vi "Read Timeout Message Priority.vi"(8 "error in (no error)":errorcluster, 11 "IEventHandler in":refnum<class "IEventHandler.lvclass">) -> (0 "error out":errorcluster, 2 "Timeout Message Priority":T1=enum."Normal", 3 "IEventHandler out":refnum<class "IEventHandler.lvclass">)   [LabVIEW 2015, in "ActorEvents.lvlib" / "IEventHandler.lvclass"]
uses:
  IEventHandler.lvclass
  <vilib>/ActorFramework/Message Enqueuer/Message Priority.ctl
  IEventHandler.lvclass/IEventHandler.ctl
  <vilib>/ActorFramework/Message Enqueuer/Message Enqueuer.lvclass
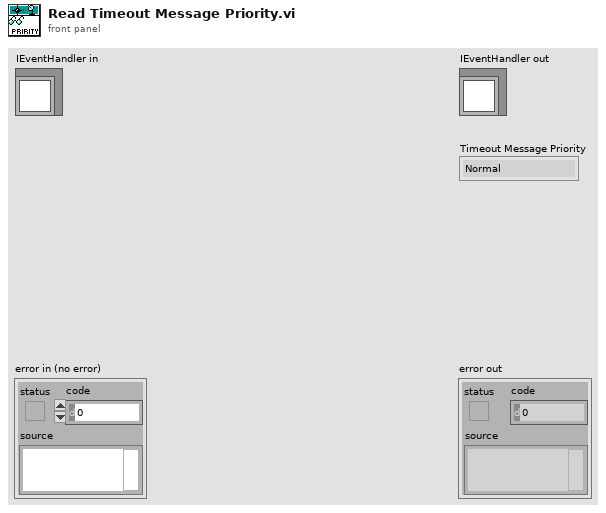
[diagram p1: front panel]
types:
  T1 = typedef "Actor Framework.lvlib/Message Enqueuer.lvclass/Message Priority.ctl" = enum16{"Low", "Normal", "High"}
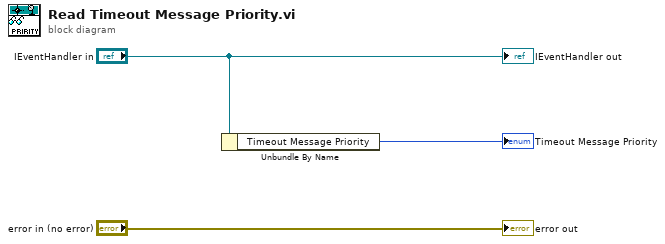
[diagram p0: block diagram]
diagram:
  n1 = Unbundle By Name("IEventHandler in") -> ("Timeout Message Priority"=→"Timeout Message Priority":T1)
  "error out" <- "error in (no error)"
  "IEventHandler out" <- "IEventHandler in"
